vi "Configure External Signal Source.vi"(0 "VISA resource name":refnum<visa-resource-name>, 1 "Divisor (1)":i32=1, 2 "Offset (0.0)":dbl format="%^.3g", 3 "Start (0.0)":dbl format="%^.3g", 4 "Stop (0.0)":dbl format="%^.3g", 5 "error in (no error)":errorcluster, 6 "Channel (1)":i32=1, 7 "Power Slope State (F: Disabled)":bool, 8 "Control State (F: Disabled)":bool, 9 "Power Level (-10.0)":dbl=-10.0 format="%^.3g", 10 "Frequency Offset State (F: Disabled)":bool, 11 "Power Slope (0.0)":dbl format="%^.3g", 12 "Multiplier (0)":i32) -> (14 "VISA resource name out":refnum<visa-resource-name>, 19 "error out":errorcluster)   [LabVIEW 2022 SP3, in "Agilent ENA Series.lvlib"]
doc: "Sets active channel and trace and configures parameters of active trace.\n\n<b>Note:</b>\nThis VI is not supported by the E5063A, E5080A and E5080B."
uses:
  <instrlib>/Agilent ENA Series/Agilent ENA Series.lvlib
panel:
  # "Note:\nThis VI is not supported by the E5063A, E5080A and E5080B."
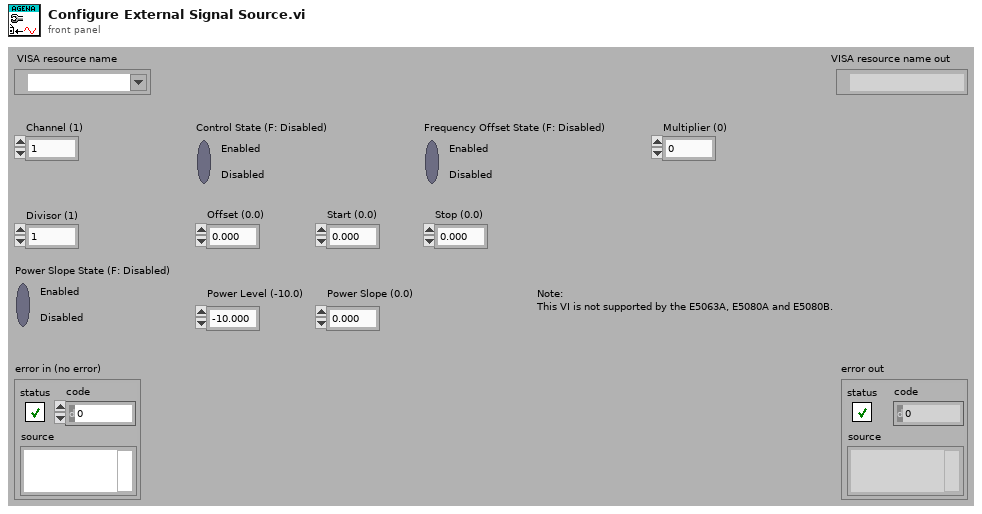
[diagram p1: front panel]
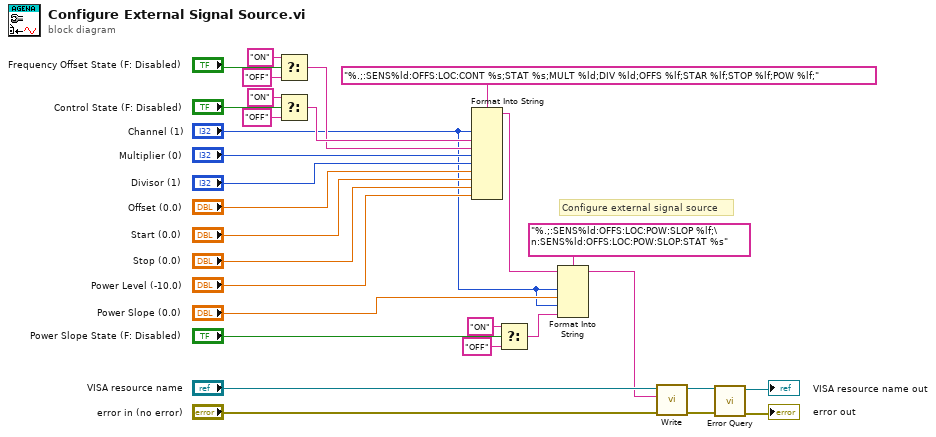
[diagram p0: block diagram]
diagram:
  # "Configure external signal source"
  n1 = Select(t="ON", s="Frequency Offset State (F: Disabled)", f="OFF") -> (s? t:f=w18:string)
  n2 = Select(t="ON", s="Control State (F: Disabled)", f="OFF") -> (s? t:f=w22:string)
  n3 = Format Into String(format string="%.;:SENS%ld:OFFS:LOC:CONT %s;STAT %s;MULT %ld;DIV %ld;OFFS %lf;STAR %lf;STOP %lf;POW %lf;", "Channel (1)", w22, w18, "Multiplier (0)", "Divisor (1)", "Offset (0.0)", "Start (0.0)", "Stop (0.0)", "Power Level (-10.0)") -> (resulting string=w23:string)  [unwired: 2 in, 1 out]
  n4 = Select(t="ON", s="Power Slope State (F: Disabled)", f="OFF") -> (s? t:f=w6:string)
  n5 = Format Into String(format string="%.;:SENS%ld:OFFS:LOC:POW:SLOP %lf;\n:SENS%ld:OFFS:LOC:POW:SLOP:STAT %s", initial string=w23, "Channel (1)", "Power Slope (0.0)", "Channel (1)", w6) -> (resulting string=w5:string)  [unwired: 1 in, 1 out]
  n6 = call <instrlib>:"Write.vi"("error in (no error)"="error in (no error)", "String ()"=w5, "VISA resource name"="VISA resource name") -> ("error out"=w3:errorcluster, "VISA resource name out"=w4:refnum<visa-resource-name>)  [unwired: 6 in, 1 out]
  n7 = call <instrlib>:"Error Query.vi"("error in (no error)"=w3, "VISA resource name"=w4) -> ("error out"=→"error out":errorcluster, "VISA resource name out"=→"VISA resource name out":refnum<visa-resource-name>)  [unwired: 6 in, 2 out]
